vi "Top_Level_Control_Cavities_v00_stripped.vi"() -> ()   [LabVIEW 2010]
doc: "Provides the user Interface for `Cavities_FPGA_v00.vi', which scans and locks 4 cavities."
uses:
  Strict Type Defs/Control GUI v01.ctl
  Strict Type Defs/Slider and display.ctl
  Strict Type Defs/I16 white control.ctl
  Strict Type Defs/PII Gains.ctl
  Strict Type Defs/I2 gain slider.ctl
  Strict Type Defs/Thresh slider.ctl
  Strict Type Defs/Lock or Hold.ctl
  Strict Type Defs/Scan Freq Slider.ctl
  Strict Type Defs/DC polarity.ctl
  Strict Type Defs/Gains negative vertical.ctl
  <vilib>/userDefined/High Color/nirio_resource_hc.ctl
  Strict Type Defs/Scope and Safety.ctl
  Strict Type Defs/Hold All.ctl
  Strict Type Defs/Cavity Extras.ctl
  Strict Type Defs/Pre-Offset.ctl
  Strict Type Defs/Lock Select 4.ctl
  <vilib>/rvi/interface/nirviOpenFPGA/nirviOpenFPGA.xnode
  FPGA Bitfiles/PIIphaselocks_FPGATarget_CavitiesFPGAv00_CFD336AA.lvbitx
  <vilib>/rvi/ClientSDK/nirviWhatTheDeviceIsDoing.ctl
  <vilib>/rvi/interface/nirviReadWriteControl/nirviReadWriteControl.xnode
  <vilib>/rvi/interface/common/niFpgaNodeNameForErrorReporting.ctl
  <vilib>/rvi/errors/niLvFpgaWhatHappensToTopLevelVI.ctl
  <vilib>/rvi/interface/nirviMethod/nirviMethod.xnode
  <vilib>/rvi/interface/nirviCloseFPGA/nirviCloseFPGA.xnode
  <vilib>/FPGAPlugInAG/PXI-7833R/niLvFpga_Open_PXI-7833R.vi
  <vilib>/rvi/interface/common/dynamic/niFpgaDynamicAddResources.vi
  <vilib>/Utility/error.llb/Error Cluster From Error Code.vi
  <vilib>/rvi/errors/niLvFpgaAdjustHostInterfaceError.vi
  <vilib>/FPGAPlugInAG/Dynamic/niLvFpga_Close_Dynamic.vi
  NiFpgaLv.dll
panel:
  in  "Lock 4":T1
  in  "OPO A":T2={"Offset Error"=-0.004322033898305084, "Gain Error"=1, "Offset DC"=0.18926553672316412, "Gain DC"=1, "P Gain"=12, "P Bit Shift"=-7, "I Bit Shift"=-7, "I2 Bit Shift"=-27, "I Gain"=19, "I2 Gain"=0, "Lock Threshold"=66, "Lock"=FALSE, "Hold"=FALSE, "Scan Frequency"=19, "Scan Bit Shift"=-4, "DC negative"=FALSE, "Gains -ve "=FALSE} {"Scan Frequency" scale=1.0..30.0; "I2 Gain" scale=0.0..10.0; "I Gain" scale=0.0..50.0; "P Gain" scale=0.0..50.0; "Offset DC" scale=-5.0..0.5 scale format="%#_5f"; "Offset Error" scale=-0.01..0.005 scale format="%#_5f"}
  in  "OPO B":T2={"Offset Error"=-0.011977401129943503, "Gain Error"=4, "Offset DC"=1.29177966101695, "Gain DC"=1, "P Gain"=14, "P Bit Shift"=-8, "I Bit Shift"=-8, "I2 Bit Shift"=-27, "I Gain"=13, "I2 Gain"=0, "Lock Threshold"=67, "Lock"=FALSE, "Hold"=FALSE, "Scan Frequency"=10, "Scan Bit Shift"=-5, "DC negative"=TRUE, "Gains -ve "=FALSE} {"Scan Frequency" scale=1.0..30.0; "I2 Gain" scale=0.0..10.0; "I Gain" scale=0.0..50.0; "P Gain" scale=0.0..50.0; "Offset DC" scale=-5.1..3.0 scale format="%#_5f"; "Offset Error" scale format="%#_5f"}
  in  "MCC":T2={"Offset Error"=-0.006610169491525424, "Gain Error"=1, "Offset DC"=0.028813559322033905, "Gain DC"=1, "P Gain"=14, "P Bit Shift"=-8, "I Bit Shift"=-11, "I2 Bit Shift"=-27, "I Gain"=11, "I2 Gain"=0, "Lock Threshold"=20, "Lock"=FALSE, "Hold"=FALSE, "Scan Frequency"=10, "Scan Bit Shift"=-4, "DC negative"=TRUE, "Gains -ve "=TRUE} {"Scan Frequency" scale=1.0..30.0; "I2 Gain" scale=0.0..10.0; "I Gain" scale=0.0..50.0; "P Gain" scale=0.0..50.0; "Offset DC" scale=-0.1..0.2 scale format="%#_5f"; "Offset Error" scale=-0.02..0.01 scale format="%#_5f"}
  in  "Doubler":T2={"Offset Error"=-0.011581920903954804, "Gain Error"=1, "Offset DC"=-0.023163841807909608, "Gain DC"=1, "P Gain"=10, "P Bit Shift"=-7, "I Bit Shift"=-8, "I2 Bit Shift"=-27, "I Gain"=21, "I2 Gain"=0, "Lock Threshold"=12, "Lock"=FALSE, "Hold"=FALSE, "Scan Frequency"=8, "Scan Bit Shift"=-5, "DC negative"=FALSE, "Gains -ve "=FALSE} {"Scan Frequency" scale=1.0..30.0; "I2 Gain" scale=0.0..10.0; "I Gain" scale=0.0..50.0; "P Gain" scale=0.0..50.0; "Offset DC" scale=-0.1..0.1 scale format="%#_5f"; "Offset Error" scale=-0.05..0.05 scale format="%#_5f"}
  out "Locked?":T12={"OPO A"=FALSE, "OPO B"=FALSE, "MCC"=FALSE, "Doubler"=TRUE}
  in  "watertank":bool
  out "Water Tank":dbl(slide)=-0.29411764705882354 scale=-0.3..0.3
  out "Top Loop Count":i32=272090
  in  "stop":bool
  in  "Hold All":T13
  in  "Extra Controls":enum32{"Scope", "Cavity Extras", "Other"}(tab)=enum."Other"
  in  "Scope+Safety":T14={"Safety First"={"lim reset"=FALSE, "no limit"=FALSE, "pos slew rate * dt"=12, "neg slew rate * dt"=-12, "Count(Ticks)"=0}, "Scope IPs"={"Trigger Direction"=enum."minus-plus", "Trigger Delay (ms)"=0.0, "Aquisition Rate (kHz)"=4000.0, "Trigger Offset (V)"=0.0, "Scale Offset"={"Scaling"={"Error signal"=1, "Output"=0, "DC Monitor"=1, "Threshold"=1}, "Offset"={"Error Signal"=0, "Output"=0, "DC Monitor"=0, "Threshold"=0}}}}
  in  "Cavity Extras":T15={"Pre-Offset"={"OPO A"=0.0, "OPO B"=0.0, "MCC"=0.0, "Doubler"=0.0}, "Pre-Offset DC"={"OPO A"=0.0, "OPO B"=0.0, "MCC"=0.0, "Doubler"=0.0}, "I Max value"=2147483647, "I2 Max value"=0, "Scan Offset"={"OPO A"=0.0, "OPO B"=0.0, "MCC"=0.0, "Doubler"=0.0}, "Scan Ampl."={"OPO A"=1000.0, "OPO B"=1000.0, "MCC"=1000.0, "Doubler"=1000.0}, "Scan-PII thresh"={"OPO A"=100, "OPO B"=100, "MCC"=100, "Doubler"=100}, "Re-Scan thresh"={"OPO A"=1, "OPO B"=1, "MCC"=4, "Doubler"=0}}
  out "Cavities Control Loop count":i32=2147483647
  in  "Lock Monitor":T17={"OPO A"=80, "OPO B"=80, "MCC"=80, "Doubler"=0}
  out "Cavities error out":errorcluster
  in  "Loop Delays (uSec)":u32=5
  in  "Number of Elements":u32=4095
  in  "Cavities_FPGA_v00":T18="RIO0" caption="RIO Device"
  in  "Scope":T8=TRUE
  out "Scope Graph":cluster{dbl[], dbl[]}[](graph)
  # "PII Gains"
  # "Lock"
  # "Error Signal"
  # "Monitor"
  # "Scan"
  # "DC positive"
  # "PII Gains"
  # "Lock"
  # "Error Signal"
  # "Monitor"
  # "Scan"
  # "DC positive"
  # "PII Gains"
  # "Lock"
  # "Error Signal"
  # "Monitor"
  # "Scan"
  # "DC positive"
  # "PII Gains"
  # "Lock"
  # "Error Signal"
  # "Monitor"
  # "Scan"
  # "DC positive"
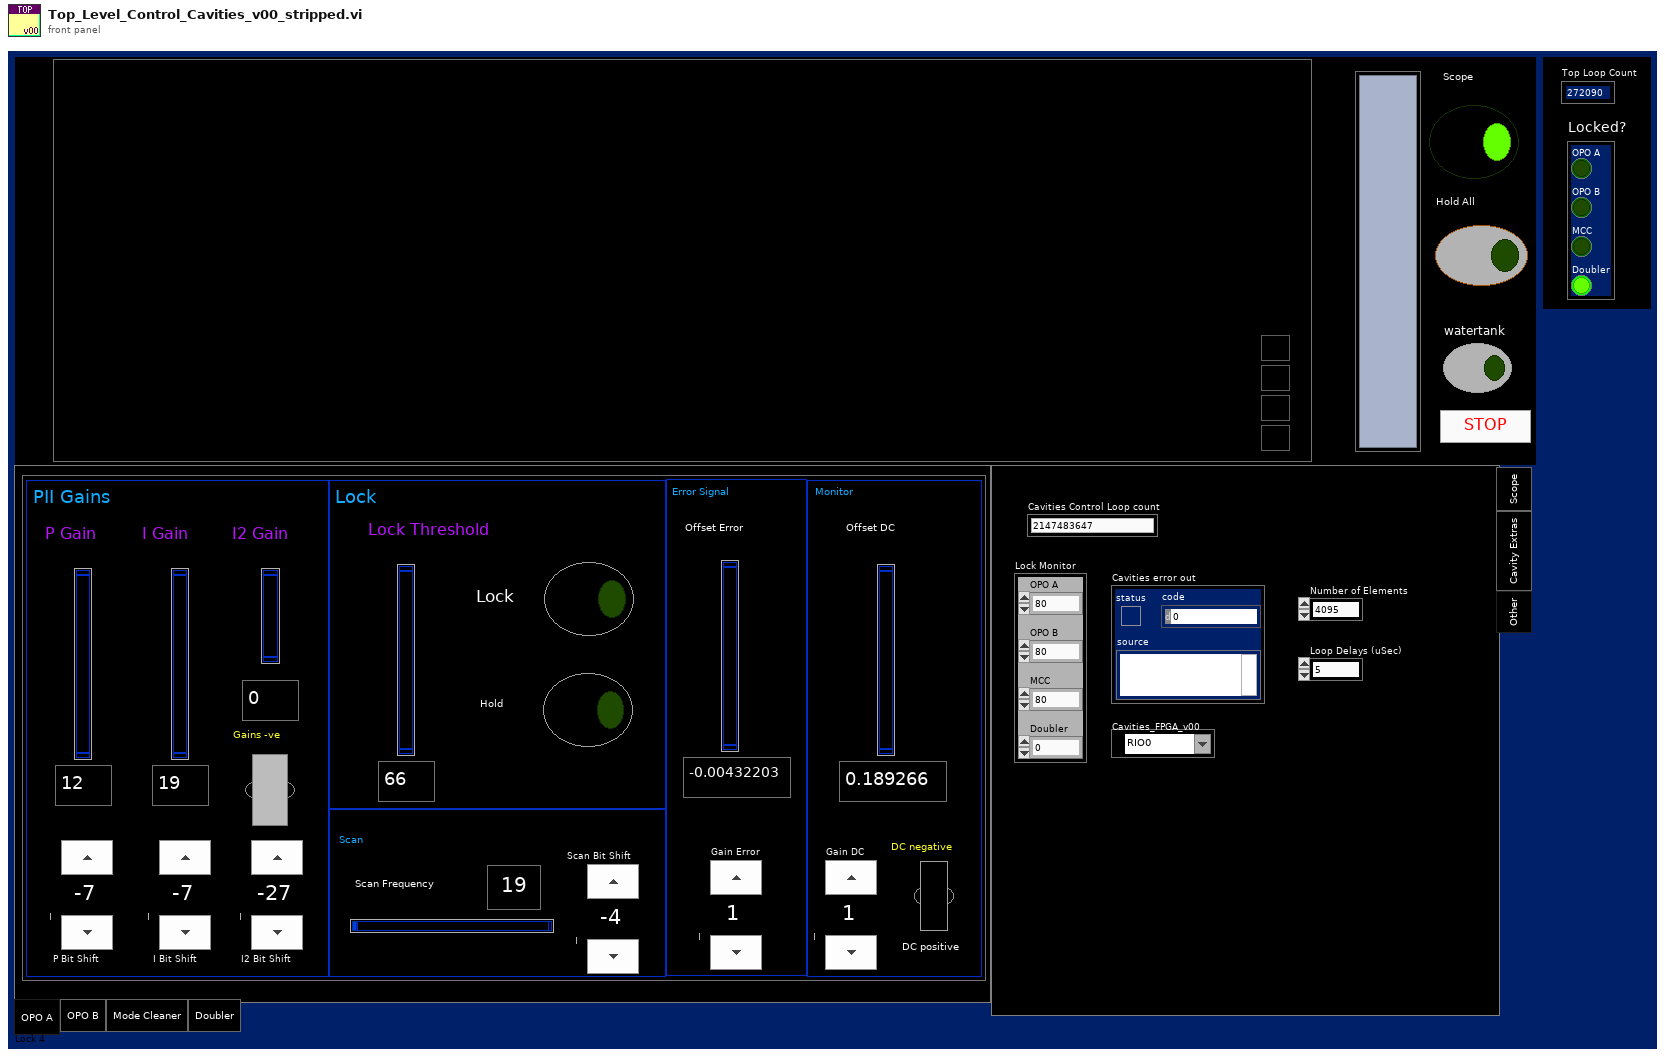
[diagram p1: front panel]
types:
  T1 = typedef "Lock Select 4.ctl" = enum32{"OPO A", "OPO B", "Mode Cleaner", "Doubler"}
  T2 = typedef "Control GUI v01.ctl" = cluster{"Offset Error":T3, "Gain Error":T4, "Offset DC":T3, "Gain DC":T4, "P Gain":T5, "P Bit Shift":T4, "I Bit Shift":T4, "I2 Bit Shift":T4, "I Gain":T5, "I2 Gain":T6, "Lock Threshold":T7, "Lock":T8, "Hold":T8, "Scan Frequency":T9, "Scan Bit Shift":T4, "DC negative":T10, "Gains -ve ":T11}
  T3 = typedef "Slider and display.ctl" = dbl
  T4 = typedef "I16 white control.ctl" = i16
  T5 = typedef "PII Gains.ctl" = i32
  T6 = typedef "I2 gain slider.ctl" = i32
  T7 = typedef "Thresh slider.ctl" = i16
  T8 = typedef "Lock or Hold.ctl" = bool
  T9 = typedef "Scan Freq Slider.ctl" = u16
  T10 = typedef "DC polarity.ctl" = bool
  T11 = typedef "Gains negative vertical.ctl" = bool
  T12 = cluster{"OPO A":bool, "OPO B":bool, "MCC":bool, "Doubler":bool}
  T13 = typedef "Hold All.ctl" = bool
  T14 = typedef "Scope and Safety.ctl" = cluster{"Safety First":cluster{"lim reset":bool, "no limit":bool, "pos slew rate * dt":i16, "neg slew rate * dt":i16, "Count(Ticks)":u32}, "Scope IPs":cluster{"Trigger Direction":enum8{"either", "minus-plus", "plus-minus"}, "Trigger Delay (ms)":dbl, "Aquisition Rate (kHz)":dbl, "Trigger Offset (V)":dbl, "Scale Offset":cluster{"Scaling":cluster{"Error signal":i16, "Output":i16, "DC Monitor":i16, "Threshold":i16}, "Offset":cluster{"Error Signal":i16, "Output":i16, "DC Monitor":i16, "Threshold":i16}}}}
  T15 = typedef "Cavity Extras.ctl" = cluster{"Pre-Offset":T16, "Pre-Offset DC":T16, "I Max value":i32, "I2 Max value":i32, "Scan Offset":T16, "Scan Ampl.":T16, "Scan-PII thresh":cluster{"OPO A":i16, "OPO B":i16, "MCC":i16, "Doubler":i16}, "Re-Scan thresh":cluster{"OPO A":i16, "OPO B":i16, "MCC":i16, "Doubler":i16}}
  T16 = typedef "Pre-Offset.ctl" = cluster{"OPO A":dbl, "OPO B":dbl, "MCC":dbl, "Doubler":dbl}
  T17 = cluster{"OPO A":i16, "OPO B":i16, "MCC":i16, "Doubler":i16}
  T18 = typedef "nirio_resource_hc.ctl" = tag
  T19 = typedef "niFpgaNodeNameForErrorReporting.ctl" = enum16{"Open FPGA VI Reference", "Read/Write Control", "Invoke Method: Abort", "Invoke Method: Acknowledge IRQ", "Invoke Method: Download", "Invoke Method: FIFO.Configure", "Invoke Method: FIFO.Read", "Invoke Method: FIFO.Start", "Invoke Method: FIFO.Stop", "Invoke Method: FIFO.Write", "Invoke Method: Reset", "Invoke Method: Run", "Invoke Method: Wait on IRQ", "Close FPGA VI Reference"}
  T20 = typedef "niLvFpgaWhatHappensToTopLevelVI.ctl" = enum16{"top level VI scripted behind XNode", "top level VI inlined behind XNode"}
  T21 = cluster{"Trigger Direction":enum8{"either", "minus-plus", "plus-minus"}, "Trigger Delay (ms)":dbl, "Aquisition Rate (kHz)":dbl, "Trigger Offset (V)":dbl, "Scale Offset":cluster{"Scaling":cluster{"Scan Scale":i16, "Scan Scale 2":i16, "Scan Scale 3":i16, "Scan Scale 4":i16}, "Offset":cluster{"Scan Offset":i16, "Scan Offset 2":i16, "Scan Offset 3":i16, "Scan Offset 4":i16}}}
  T22 = cluster{"PII In 1":cluster{"Lock":bool, "Hold":bool, "P Gain":i32, "P BS":i16, "I Gain":i32, "I BS":i16, "I2 G":i32, "I2 BS":i16, "Scan Amp":i16, "Scan Off":i16, "Scan FS":u16, "SFS BS":i16, "I Max value":i32, "I2 Max value":i32, "Scope.Offset":i16, "Trigger Direction":enum8{"either", "minus-plus", "plus-minus"}, "Scan-PII thresh":i16}, "PII In 2":cluster{"Lock":bool, "Hold":bool, "P Gain":i32, "P BS":i16, "I Gain":i32, "I BS":i16, "I2 G":i32, "I2 BS":i16, "Scan Amp":i16, "Scan Off":i16, "Scan FS":u16, "SFS BS":i16, "I Max value":i32, "I2 Max value":i32, "Scope.Offset":i16, "Trigger Direction":enum8{"either", "minus-plus", "plus-minus"}, "Scan-PII thresh":i16}, "PII In 3":cluster{"Lock":bool, "Hold":bool, "P Gain":i32, "P BS":i16, "I Gain":i32, "I BS":i16, "I2 G":i32, "I2 BS":i16, "Scan Amp":i16, "Scan Off":i16, "Scan FS":u16, "SFS BS":i16, "I Max value":i32, "I2 Max value":i32, "Scope.Offset":i16, "Trigger Direction":enum8{"either", "minus-plus", "plus-minus"}, "Scan-PII thresh":i16}, "PII In 4":cluster{"Lock":bool, "Hold":bool, "P Gain":i32, "P BS":i16, "I Gain":i32, "I BS":i16, "I2 G":i32, "I2 BS":i16, "Scan Amp":i16, "Scan Off":i16, "Scan FS":u16, "SFS BS":i16, "I Max value":i32, "I2 Max value":i32, "Scope.Offset":i16, "Trigger Direction":enum8{"either", "minus-plus", "plus-minus"}, "Scan-PII thresh":i16}, "Safety First":cluster{"lim reset":bool, "no limit":bool, "pos slew rate * dt":i16, "neg slew rate * dt":i16, "Hold All":bool, "Count(Ticks)":u32}, "Error scale":cluster{"Pre-Offset":cluster{"Pre-Offset 1":i16, "Pre-Offset 2":i16, "Pre-Offset 3":i16, "Pre-Offset 4":i16, "Pre-Offset 5":i16, "Pre-Offset 6":i16, "Pre-Offset 7":i16, "Pre-Offset 8":i16}, "Post-Offset ":cluster{"Offset 1":i16, "Offset 2":i16, "Offset 3":i16, "Offset 4":i16, "Offset 5":i16, "Offset 6":i16, "Offset 7":i16, "Offset 8":i16}, "Gains":cluster{"Gain 1":i16, "Gain 2":i16, "Gain 3":i16, "Gain 4":i16, "Gain 5":i16, "Gain 6":i16, "Gain 7":i16, "Gain 8":i16}, "Polarity DC":cluster{"False 1":bool, "False 2":bool, "False 3":bool, "False 4":bool, "DC x -1":bool, "DC x -1 2":bool, "DC x -1 3":bool, "DC x -1 4":bool}}, "Lock Thresh":cluster{"OPO A":i16, "OPO B":i16, "MCC":i16, "Doubler":i16}, "Re-Scan Thresh":cluster{"OPO A":i16, "OPO B":i16, "MCC":i16, "Doubler":i16}}
  T23 = cluster{"Trigger Direction":enum8{"either", "minus-plus", "plus-minus"}, "Delay":u32, "Aquisition Rate (Ticks)":u32, "Offset":i16, "Channel":i32, "Channel Selector":cluster{"Channel 1":i32, "Channel 2":i32, "Channel 3":i32, "Channel 4":i32}}
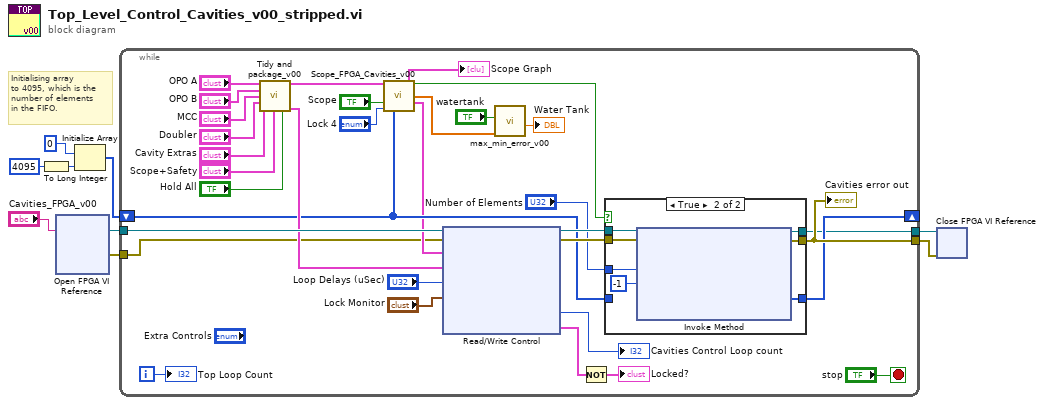
[diagram p0: block diagram]
diagram:
  # "Initialising array\nto 4095, which is the\nnumber of elements\nin the FIFO."
  n1 = To Long Integer(number=4095) -> (32bit integer=w6:i32)
  n2 = xnode "Open FPGA VI Reference"("resource name"="Cavities_FPGA_v00") -> ("FPGA VI Reference Out"=w8:refnum<k20>, "error out"=w7:errorcluster)  [unwired: 1 in]
  n3 = Initialize Array(u64 0 ("element"), w6) -> (w3:u64[])
  n4 = while {
    tunnel: w8 -> [w42]
    tunnel: w7 -> [w20]
    tunnel: [w38] -> w1
    shift-right: [w36] -> _
    shift-left: w3 -> [w26]
    tunnel: [w35] -> w2
    i -> [w40]
    stop <- "stop" stop-if-true
    n5 = call "Tidy and package_v00.vi"("OPO A"="OPO A", "OPO B"="OPO B", "MCC"="MCC", "Doubler"="Doubler", "Cavity Extras"="Cavity Extras", "Scope+Safety"="Scope+Safety", "Hold All"="Hold All") -> ("Scope IPs"=w28:T21, "Control to FPGA"=w30:T22)  [unwired: 6 in, 1 out]
    n6 = call "Scope_FPGA_Cavities_v00.vi"("Scope IPs"=w28, "Scope"="Scope", "Lock 4"="Lock 4", "Cavities Data"=w26) -> ("Scope OP Graph"=→"Scope Graph":cluster{dbl[], dbl[]}[], "Scope Cavities ON"=w13:bool, "error"=w19:dbl[], "Scope Cavities"=w23:T23)  [unwired: 8 in]
    n7 = xnode "Read/Write Control"("FPGA VI Reference In"=w42, "error in"=w20, "Scope"=w23, "Control"=w30, "Cavities Delay(uSec)"="Loop Delays (uSec)", "Lock Monitor"="Lock Monitor") -> ("FPGA VI Reference Out"=w37:refnum<k20>, "error out"=w39:errorcluster, "Control Loop count"=→"Cavities Control Loop count":i32, "Unlocked?(T=yes)"=w14:T12)
    n8 = call "max_min_error_v00.vi"("Array"=w19, "maxmin"="watertank") -> ("x+y"=→"Water Tank":dbl)  [unwired: 7 in, 2 out]
    n9 = Not(x=w14) -> (.not. x?=→"Locked?":T12)
    n10 = case shown="True" w13 {
      tunnel: w39 -> [w45 w52]
      tunnel: [w45 w51] -> w38
      tunnel: w37 -> [w44 w50]
      tunnel: [w44 w49] -> w35
      tunnel: [w43 w48] -> w36
      tunnel: w26 -> [w43 _]
      tunnel: "Number of Elements" -> [_ w46]
      frame False {
      }
      frame True {
        n11 = xnode "Invoke Method"("FPGA VI Reference In"=w50, "error in"=w52, "Number of Elements"=w46, "Timeout (ms)"=-1) -> ("FPGA VI Reference Out"=w49:refnum<k20>, "error out"=w51:errorcluster, "Data"=w48:u64[])  [unwired: 1 out]
      }
    }
    "Cavities error out" <- w38
    "Top Loop Count" <- w40
  }
  n12 = xnode "Close FPGA VI Reference"("FPGA VI Reference In"=w2, "error in"=w1) -> ()  [unwired: 1 out]
